vi "(Sub) System State Check.vi"(8 "error in (no error)":errorcluster caption="에러 입력(에러 없음)", 9 "Read  Mode":string, 10 "Read HV State":string, 11 "Read System State":string) -> (0 "error out":errorcluster caption="에러 출력", 2 "시스템 비정상?":bool, 3 "Out System State":T1)   [LabVIEW 2017]
uses:
  Controls/(Ctrl) System State.ctl
panel:
  # "Group.1"
  # "Voltage Mode On"
  # "Current Mode On"
  # "HV On"
  # "Regulator Error"
  # "Local Mode"
  # "System Fault"
  # "Adjustable Overload Fault"
  # "Over Temperature"
  # "Arc Fault"
  # "Over Power"
  # "Over Current"
  # "Over Voltage Fault"
  # "HV Inhibited"
  # "Interlock open"
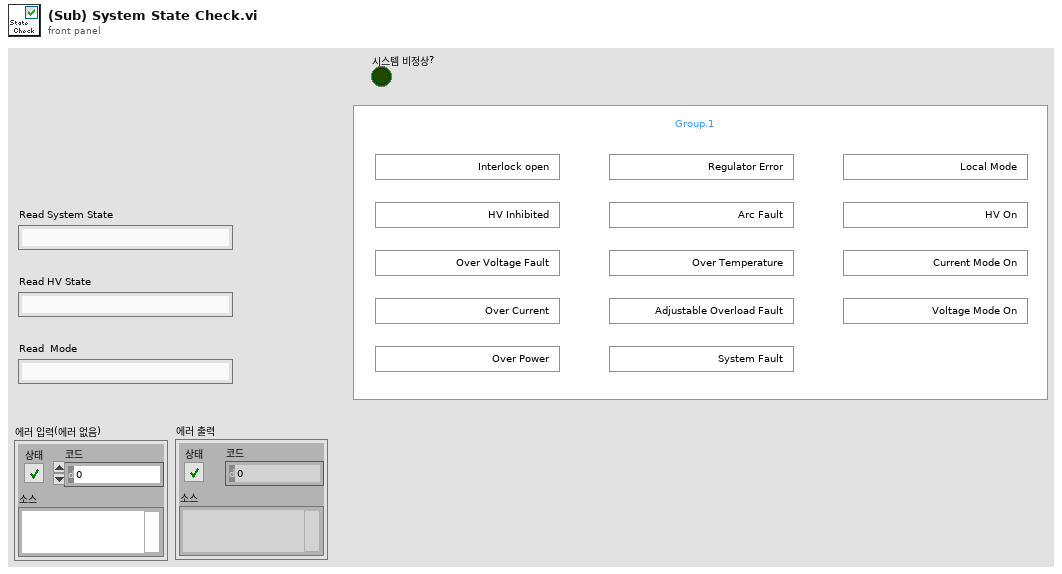
[diagram p1: front panel]
types:
  T1 = typedef "(Ctrl) System State.ctl" = cluster{"Interlock open":bool, "HV Inhibited":bool, "Over Voltage Fault":bool, "Over Current":bool, "Over Power":bool, "Regulator Error":bool, "Arc Fault":bool, "Over Temperature":bool, "Adjustable Overload Fault":bool, "System Fault":bool, "Remote Mode":bool, "HV On":bool, "Current Mode On":bool, "Voltage Mode On":bool}
  T2 = cluster{"[0]":bool, "[1]":bool, "[2]":bool, "[3]":bool, "[4]":bool, "[5]":bool, "[6]":bool, "[7]":bool, "[8]":bool, "[9]":bool, "[10]":bool, "[11]":bool, "[12]":bool, "[13]":bool}
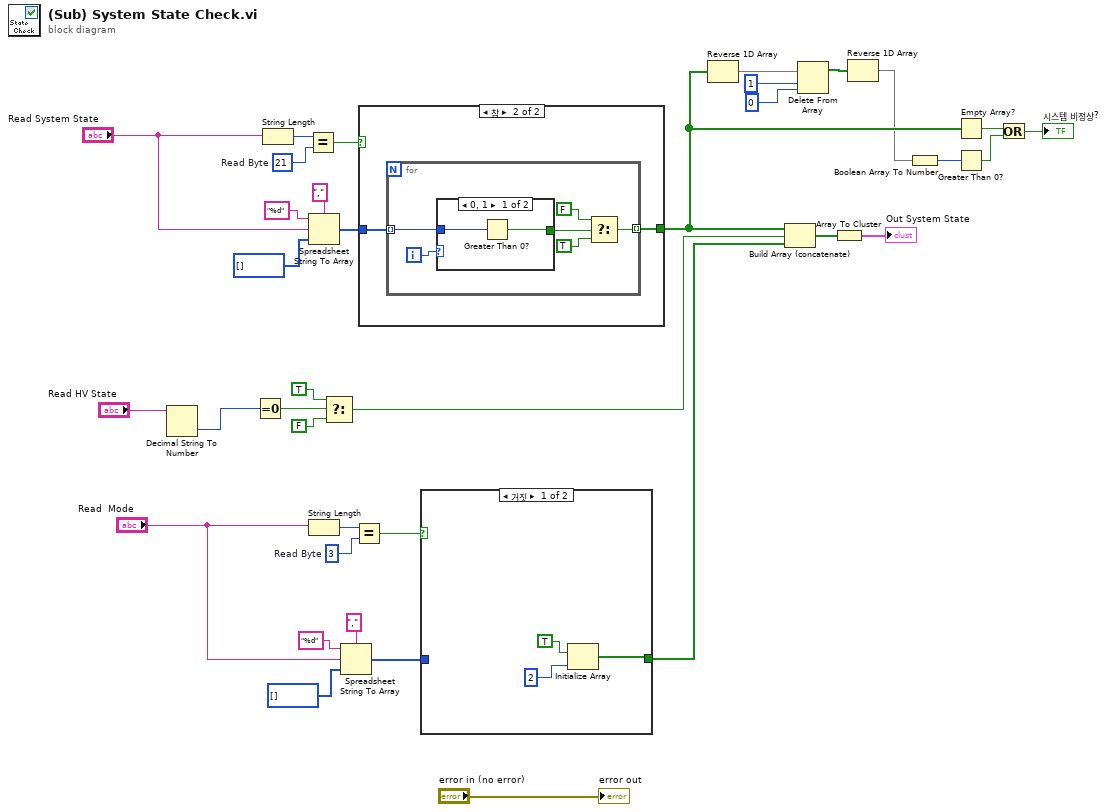
[diagram p0: block diagram]
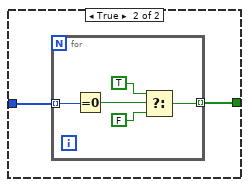
[diagram p2: hidden frame]
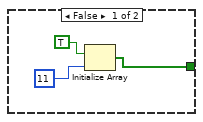
[diagram p3: hidden frame]
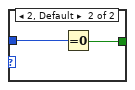
[diagram p4: hidden frame]
diagram:
  w9 = 3  # Read Byte
  w35 = 21  # Read Byte
  n1 = Decimal String To Number(string="Read HV State") -> (number=w25:i32)  [unwired: 2 in, 1 out]
  n2 = Equal To 0?(x=w25) -> (x = 0?=w28:bool)
  n3 = String Length(string="Read System State") -> (length=w36:i32)
  n4 = Equal?(x=w36, y=w35) -> (x = y?=w34:bool)
  n5 = Spreadsheet String To Array(delimiter (Tab)="," ("구분 문자 (탭)"), format string="%d" ("포맷 문자열"), spreadsheet string="Read System State", array type (2D Dbl)=i32[] []) -> (array=w29:i32[])
  n6 = String Length(string="Read  Mode") -> (length=w10:i32)
  n7 = Select(t=TRUE, s=w28, f=FALSE) -> (s? t:f=w19:bool)
  n8 = Spreadsheet String To Array(delimiter (Tab)="," ("구분 문자 (탭)"), format string="%d" ("포맷 문자열"), spreadsheet string="Read  Mode", array type (2D Dbl)=i32[] []) -> (array=w20:i32[])
  n9 = Equal?(x=w10, y=w9) -> (x = y?=w7:bool)
  n10 = case shown="참" w34 {
    tunnel: w29 -> [_ w41]
    tunnel: [w38 w40] -> w4
    frame False {
      n11 = Initialize Array(TRUE, 11 ("차원 크기")) -> (w38:bool[])
    }
    frame True {
      n12 = for {
        tunnel: w41 -> [w47] mode=indexing
        tunnel: [w43] -> w40 mode=indexing
        i -> [w42]
        n13 = case shown="0, 1" w42 {
          tunnel: w47 -> [w49 w51]
          tunnel: [w48 w50] -> w44
          frame 0, 1 {
            n14 = Greater Than 0?(x=w49) -> (x > 0?=w48:bool)
          }
          frame 2, Default {
            n15 = Equal To 0?(x=w51) -> (x = 0?=w50:bool)
          }
        }
        n16 = Select(t=FALSE, s=w44, f=TRUE) -> (s? t:f=w43:bool)
      }
    }
  }
  n17 = case shown="거짓" w7 {
    tunnel: w20 -> [_ w56]
    tunnel: [w52 w55] -> w18
    frame False {
      n18 = Initialize Array(TRUE, 2 ("차원 크기")) -> (w52:bool[])
    }
    frame True {
      n19 = for {
        tunnel: w56 -> [w58] mode=indexing
        tunnel: [w57] -> w55 mode=indexing
        n20 = Equal To 0?(x=w58) -> (x = 0?=w61:bool)
        n21 = Select(t=TRUE, s=w61, f=FALSE) -> (s? t:f=w57:bool)
      }
    }
  }
  n22 = Reverse 1D Array(array=w4) -> (reversed array=w3:bool[])
  n23 = Build Array (concatenate)(w4, w19, w18) -> (w17:bool[])
  n24 = Delete From Array(array=w3, length=1 ("인덱스"), index=0 ("길이")) -> (array with subset deleted=w1:bool[])  [unwired: 1 out]
  n25 = Array To Cluster(array=w17) -> (cluster=→"Out System State":T2)
  n26 = Reverse 1D Array(array=w1) -> (reversed array=w2:bool[])
  n27 = Boolean Array To Number(Boolean array=w2) -> (number=w16:u32)
  n28 = Empty Array?(array=w4) -> (empty?=w15:bool)
  n29 = Greater Than 0?(x=w16) -> (x > 0?=w14:bool)
  n30 = Or(x=w15, y=w14) -> (x .or. y?=→"시스템 비정상?":bool)
  "error out" <- "error in (no error)"
